vi "Format Double Numeric.vi"(1 "value":dbl) -> (0 "String":string)   [LabVIEW 2020, in "Astemes_CSVReportPlugin.lvlib" / "TestStand Result Handler.lvclass"]
uses:
  TestStand Result Handler.lvclass
  TestStand Result Handler.lvclass/TestStand Result Handler.ctl
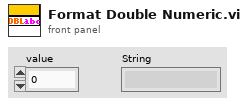
[diagram p1: front panel]
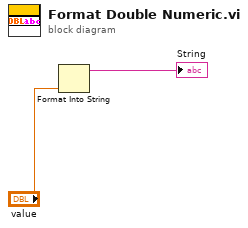
[diagram p0: block diagram]
diagram:
  n1 = Format Into String("value") -> (resulting string=→"String":string)  [unwired: 3 in, 1 out]
